vi "GET_GPIO_n.vi"(2 "execute":bool, 11 "error in (no error)":errorcluster) -> (4 "function return":string, 8 "uLPtr":u32[](array[numeric]), 15 "error out":errorcluster)   [LabVIEW 2013, in "ZBOX_IS.lvlib"]
uses:
  <instrlib>/ZBOX_IS/ZBOX_IS.lvlib
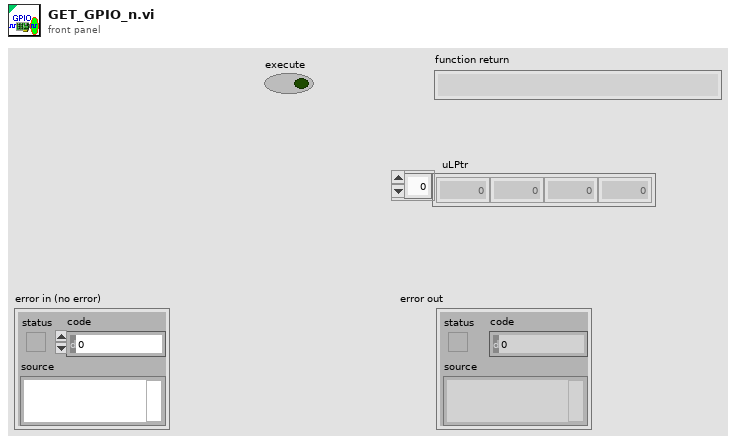
[diagram p1: front panel]
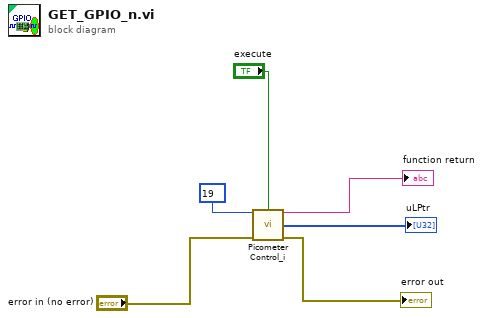
[diagram p0: block diagram]
diagram:
  n1 = call <instrlib>:"Picometer Control_i.vi"("Cmd"=u8 19, "execute"="execute", "error in (no error)"="error in (no error)") -> ("function return"=→"function return":string, "uLPtr"=→"uLPtr":u32[], "error out"=→"error out":errorcluster)  [unwired: 8 in, 2 out]
